vi "Write Status.vi"(8 "error in (no error)":errorcluster, 10 "status":T1 {"duration" format="%d us"}, 11 "status pointer in":refnum<class "Status.lvclass">) -> (0 "error out":errorcluster, 3 "status pointer out":refnum<class "Status.lvclass">)   [LabVIEW 2017, in "DSF Core.lvlib" / "Status.lvclass"]
uses:
  Status.lvclass
  C:/Git/DSF/LabVIEW-Memory/Source/Classes/Pointer/Pointer.lvclass
  Status/Status Data.ctl
  LabVIEW-Memory/Source/Classes/Pointer/Pointer.lvclass
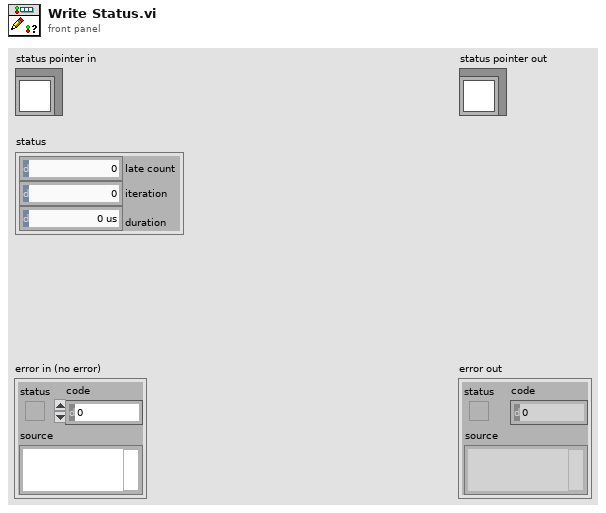
[diagram p1: front panel]
types:
  T1 = typedef "DSF Core.lvlib/Status.lvclass/Status Data.ctl" = cluster{"late count":u64, "iteration":u64, "duration":u32}
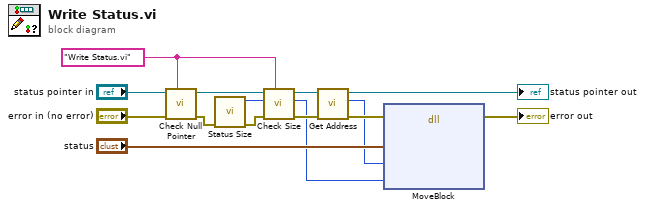
[diagram p0: block diagram]
diagram:
  w5 = "Write Status.vi" ("source vi name")
  n1 = call "Check Null Pointer.vi"("source vi name"=w5, "error in (no error)"="error in (no error)", "Pointer in"="status pointer in") -> ("error out"=w9:errorcluster, "Pointer out"=w10:refnum<class "Status.lvclass">)  [unwired: 7 in]
  n2 = call "Status Size.vi"("error in (no error)"=w9) -> ("error out"=w11:errorcluster, "size"=w8:u64)  [unwired: 9 in]
  n3 = call "Check Size.vi"("source vi name"=w5, "error in (no error)"=w11, "required size"=w8, "Pointer in"=w10) -> ("error out"=w4:errorcluster, "required size out"=w1:u64, "Pointer out"=w6:refnum<class "Status.lvclass">)  [unwired: 5 in]
  n4 = call "Get Address.vi"("Pointer in"=w6) -> ("address"=w2:u64, "Pointer out"=→"status pointer out":refnum<class "Status.lvclass">)  [unwired: 9 in]
  n5 = dll-call lib="LabVIEW" fn="MoveBlock"(error in=w4, "src"="status", "dst"=w2, "size"=w1) -> (error out=→"error out":errorcluster)  [unwired: 6 in, 1 out]
